vi "RFmx_Continuous_MeasureTest.vi"() -> ()   [LabVIEW 2014]
uses:
  <vilib>/RFmx/RFInstr/mx/RFmxInstr.llb/RFmxInstr Build Signal String.vi
  <vilib>/RFmx/SpecAn/mx/RFmxSpecAn.llb/RFmxSpecAn Configure Digital Edge Trigger.vi
panel:
  out "ExT":dbl format="%#_6p"
  in  "Stop Button":bool
  # "[ RFmx  Meas Test ]"
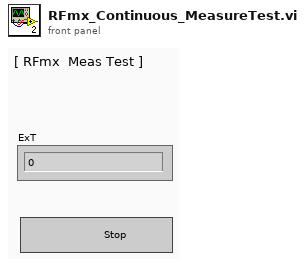
[diagram p1: front panel]
types:
  T1 = typedef "Message_Queues.ctl" = cluster{"RFSG_QTx":refnum<queue>, "RFSG_QRx":refnum<queue>, "RFSA_QTx":refnum<queue>, "RFSA_QRx":refnum<queue>, "SysLog":refnum<queue>, "RFSA_Data":refnum<queue>, "RFmx_QTx":refnum<queue>, "RFmx_QRx":refnum<queue>, "RFmx_Data":refnum<queue>}
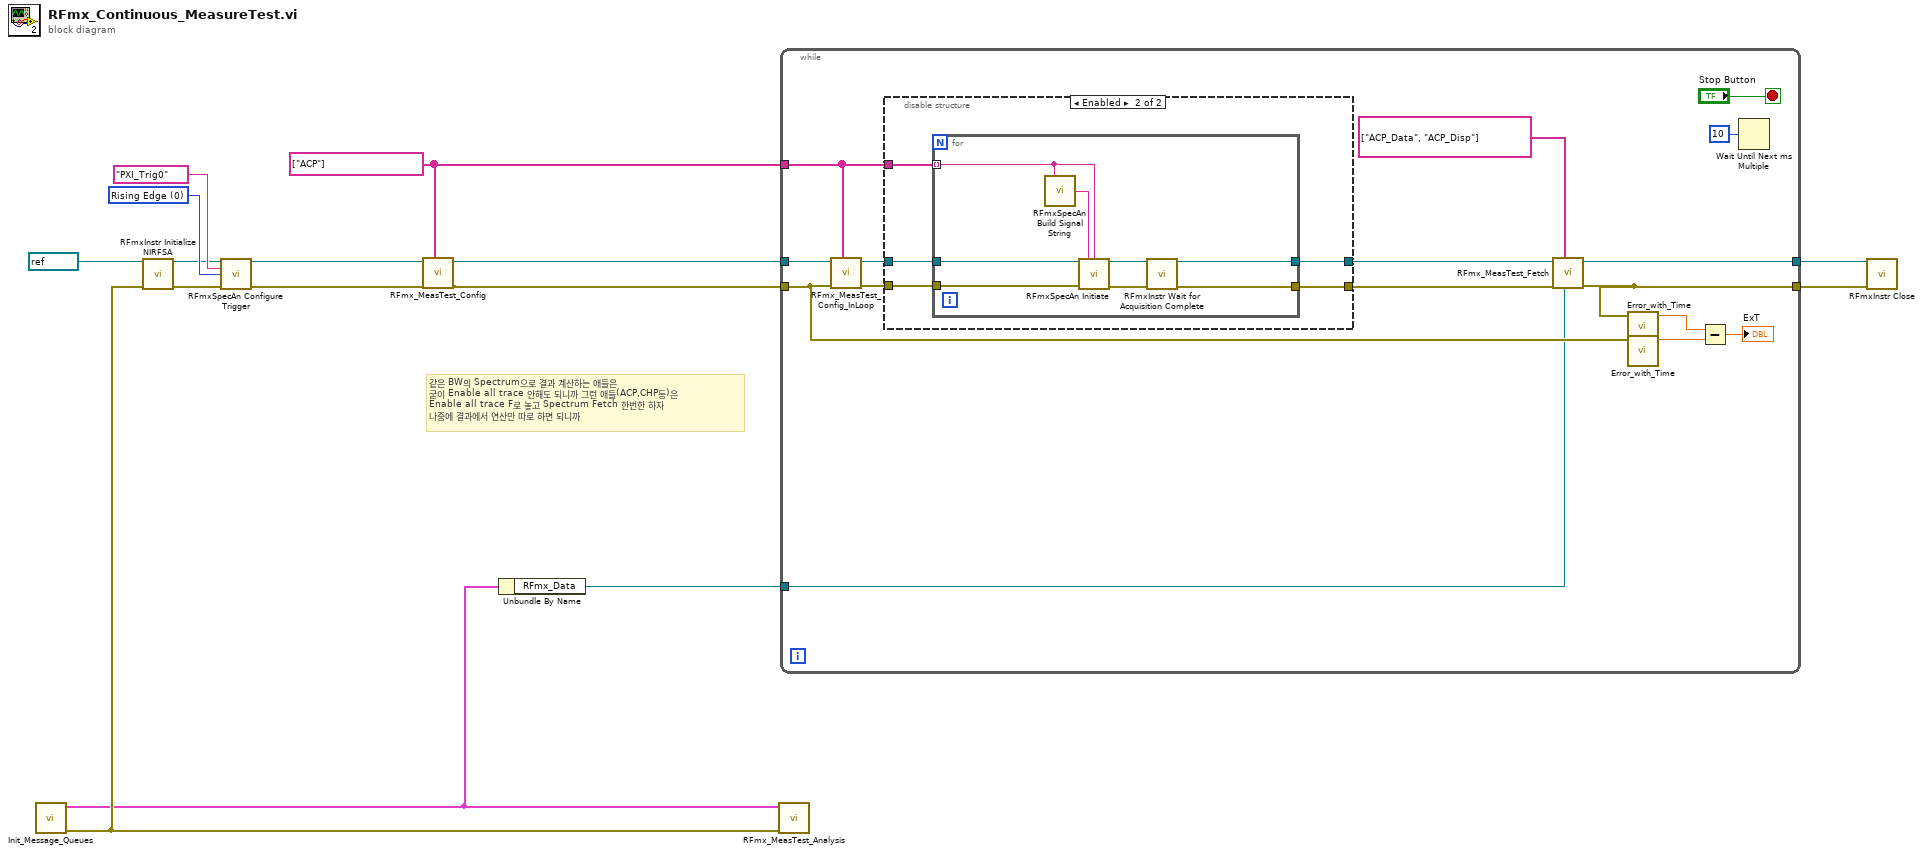
[diagram p0: block diagram]
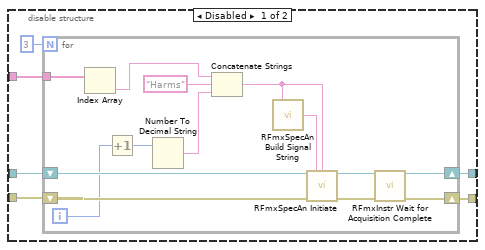
[diagram p2: hidden frame]
diagram:
  w5 = string[] ["ACP"]
  w13 = 0 items=["Rising Edge", "Falling Edge"] ("Digital Edge")
  # "같은 BW의 Spectrum으로 결과 계산하는 애들은\n굳이 Enable all trace 안해도 되니까 그런 애들(ACP,CHP등)은\nEnable all trace F로 놓고 Spectrum Fetch 한번한 하자\n나중에 결과에서 연산만 따로 하면 되니까"
  n1 = call "Init_Message_Queues.vi"() -> ("error out"=w8:errorcluster, "Queue_Out"=w7:T1)  [unwired: 10 in]
  n2 = call <vilib>:"RFmxInstr Initialize NIRFSA.vi"("Resource Name"=refnum<k15> "VST", "error in (no error)"=w8) -> ("Instrument Handle Out"=w2:refnum<k21>, "error out"=w1:errorcluster)  [unwired: 11 in, 1 out]
  n3 = call-poly <vilib>:"RFmxSpecAn Configure Trigger.vi"("Instrument Handle In"=w2, "Digital Edge Source"="PXI_Trig0", "Digital Edge"=w13, "error in (no error)"=w1) -> ("Instrument Handle Out"=w9:refnum<k21>, "error out"=w10:errorcluster)  [unwired: 10 in]
  n4 = call "RFmx_MeasTest_Config.vi"("Meas_Type"=w5, "error in (no error)"=w10, "Instrument Handle in"=w9) -> ("error out"=w3:errorcluster, "Instrument Handle out"=w4:refnum<k21>)  [unwired: 7 in]
  n5 = Unbundle By Name(w7) -> ("RFmx_Data"=w6:refnum<queue>)
  n6 = call "RFmx_MeasTest_Analysis.vi"("error in (no error)"=w8, "Message_Queues"=w7) -> ()  [unwired: 9 in, 1 out]
  n7 = while {
    tunnel: w4 -> [w26]
    tunnel: w3 -> [w24]
    tunnel: [w18] -> w11
    tunnel: [w17] -> w12
    tunnel: w6 -> [w20]
    tunnel: w5 -> [w16]
    stop <- "Stop Button" stop-if-true
    n8 = call "RFmx_MeasTest_Config_InLoop.vi"("Meas_Type"=w16, "error in (no error)"=w24, "Instrument Handle in"=w26) -> ("error out"=w23:errorcluster, "Instrument Handle out"=w25:refnum<k21>)  [unwired: 7 in]
    n9 = disable-structure shown="Enabled" {
      disable-tunnel: w25 -> [w37 w56]
      disable-tunnel: w23 -> [w36 w55]
      disable-tunnel: [w35 w53] -> w22
      disable-tunnel: [w34 w54] -> w21
      disable-tunnel: w16 -> [w33 w52]
      frame Disabled {
        n10 = for {
          N: 3 -> [_]
          shift-right: [w45] -> w35
          shift-left: w37 -> [w51]
          shift-right: [w46] -> w34
          shift-left: w36 -> [w50]
          tunnel: w33 -> [w41]
          i -> [w39]
          n11 = Index Array(array=w41) -> (element=w40:string)  [unwired: 1 in]
          n12 = Increment(x=w39) -> (x+1=w38:i32)
          n13 = Number To Decimal String(number=w38) -> (decimal integer string=w43:string)  [unwired: 1 in]
          n14 = Concatenate Strings(w40, "Harms", w43) -> (w42:string)
          n15 = call <vilib>:"RFmxSpecAn Build Signal String.vi"("Signal Name"=w42) -> ("Selector String"=w49:string)  [unwired: 14 in]
          n16 = call <vilib>:"RFmxSpecAn Initiate.vi"("Instrument Handle In"=w51, "Selector String"=w49, "Result Name"=w42, "error in (no error)"=w50) -> ("Instrument Handle Out"=w48:refnum<k21>, "error out"=w47:errorcluster)  [unwired: 9 in, 1 out]
          n17 = call <vilib>:"RFmxInstr Wait for Acquisition Complete.vi"("Instrument Handle In"=w48, "error in (no error)"=w47) -> ("Instrument Handle Out"=w45:refnum<k21>, "error out"=w46:errorcluster)  [unwired: 12 in]
        }
      }
      frame Enabled {
        n18 = for {
          tunnel: w56 -> [w61]
          tunnel: w55 -> [w60]
          tunnel: [w59] -> w54
          tunnel: [w58] -> w53
          tunnel: w52 -> [w57] mode=indexing
          n19 = call <vilib>:"RFmxSpecAn Build Signal String.vi"("Signal Name"=w57) -> ("Selector String"=w64:string)  [unwired: 14 in]
          n20 = call <vilib>:"RFmxSpecAn Initiate.vi"("Instrument Handle In"=w61, "Selector String"=w64, "Result Name"=w57, "error in (no error)"=w60) -> ("Instrument Handle Out"=w63:refnum<k21>, "error out"=w62:errorcluster)  [unwired: 9 in, 1 out]
          n21 = call <vilib>:"RFmxInstr Wait for Acquisition Complete.vi"("Instrument Handle In"=w63, "error in (no error)"=w62) -> ("Instrument Handle Out"=w58:refnum<k21>, "error out"=w59:errorcluster)  [unwired: 12 in]
        }
      }
    }
    n22 = call "RFmx_MeasTest_Fetch.vi"("RFmx_Data"=w20, "Meas_Type"=string[] ["ACP_Data", "ACP_Disp"], "error in (no error)"=w21, "Instrument Handle in"=w22) -> ("error out"=w17:errorcluster, "Instrument Handle out"=w18:refnum<k21>)  [unwired: 6 in]
    n23 = call "Error_with_Time.vi"("error in (no error)"=w17) -> ("relative seconds"=w29:dbl)  [unwired: 10 in]
    n24 = call "Error_with_Time.vi"("error in (no error)"=w24) -> ("relative seconds"=w28:dbl)  [unwired: 10 in]
    n25 = Subtract(x=w29, y=w28) -> (x-y=→"ExT":dbl)
    n26 = Wait Until Next ms Multiple(millisecond multiple=u32 10) -> ()  [unwired: 1 out]
  }
  n27 = call <vilib>:"RFmxInstr Close.vi"("Instrument Handle In"=w11, "error in (no error)"=w12) -> ()  [unwired: 13 in, 1 out]
